vi "LCM.vi"(10 "y":i64, 11 "x":i64) -> (3 "lcm(x,y)":i64)   [LabVIEW 2023]
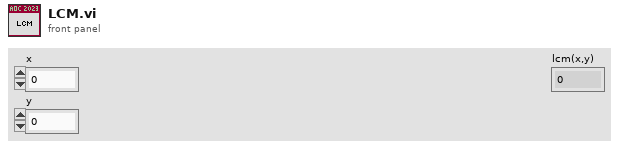
[diagram p1: front panel]
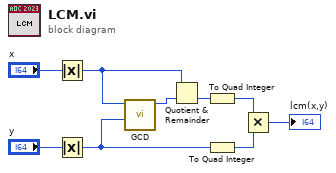
[diagram p0: block diagram]
diagram:
  n1 = Absolute Value(x="x") -> (abs(x)=w3:i64)
  n2 = Absolute Value(x="y") -> (abs(x)=w2:i64)
  n3 = call "GCD.vi"("y"=w2, "x"=w3) -> ("gcd(x,y)"=w1:i64)  [unwired: 9 in]
  n4 = Quotient & Remainder(x=w3, y=w1) -> (floor(x/y)=w7:i64)  [unwired: 1 out]
  n5 = To Quad Integer(1:w7) -> (0:w4:i64)
  n6 = To Quad Integer(1:w2) -> (0:w5:i64)
  n7 = Multiply(x=w4, y=w5) -> (x*y=→"lcm(x,y)":i64)
